vi "Read Data.vi"(8 "error in (no error)":errorcluster, 10 "Count":i32, 11 "FileStream in":refnum<class "FileStream.lvclass">) -> (0 "error out":errorcluster, 2 "Data":string, 3 "FileStream out":refnum<class "FileStream.lvclass">)   [LabVIEW 2020, in "IO.lvlib" / "FileStream.lvclass"]
uses:
  FileStream.lvclass
  FileStream.lvclass/FileStream.ctl
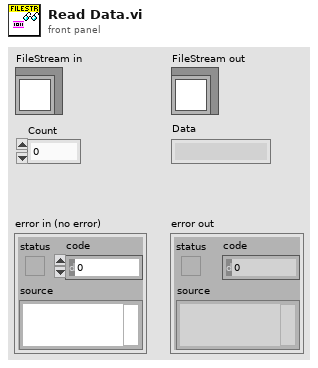
[diagram p1: front panel]
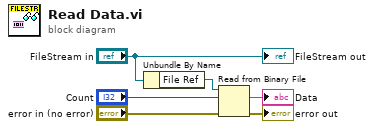
[diagram p0: block diagram]
diagram:
  n1 = Unbundle By Name("FileStream in") -> ("File Ref"=w4:refnum<file>)
  n2 = Read from Binary File(8:"error in (no error)", 10:"Count", 11:w4) -> (0:→"error out":errorcluster, 2:→"Data":string)  [unwired: 3 in, 2 out]
  "FileStream out" <- "FileStream in"
